vi "File.Convert CSV Item to String.vi"(11 "String":string) -> (3 "String Out":string)   [LabVIEW 2024, in "EQMF.lvlib" / "File Utils.lvlib"]
uses:
  File Utils.lvlib
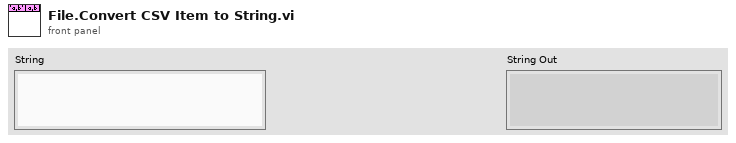
[diagram p1: front panel]
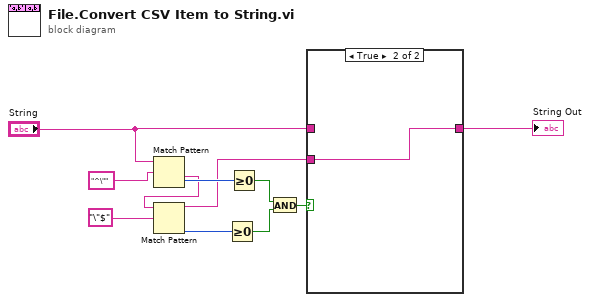
[diagram p0: block diagram]
diagram:
  n1 = Match Pattern(string="String", regular expression="^\"") -> (after substring=w2:string, offset past match=w11:i32)  [unwired: 1 in, 2 out]
  n2 = Match Pattern(string=w2, regular expression="\"$") -> (before substring=w1:string, offset past match=w10:i32)  [unwired: 1 in, 2 out]
  n3 = Greater Or Equal To 0?(x=w10) -> (x >= 0?=w8:bool)
  n4 = Greater Or Equal To 0?(x=w11) -> (x >= 0?=w9:bool)
  n5 = And(x=w9, y=w8) -> (x .and. y?=w7:bool)
  n6 = case shown="True" w7 {
    tunnel: "String" -> [w12 _]
    tunnel: [w12 w13] -> w5
    tunnel: w1 -> [_ w13]
    frame False {
    }
    frame True {
    }
  }
  "String Out" <- w5
